vi "New Exchanges.vi"(8 "error in (no error)":errorcluster caption="entrée d'erreur (pas d'erreur)", 10 "initial dictionary (empty)":cluster{"key":variant, "value":variant}[](array[cluster]), 11 "Exchanges en entrée":refnum<class "Exchanges.lvclass"> caption="DNL_LabVIEW Object in") -> (0 "error out":errorcluster caption="sortie d'erreur", 3 "Exchanges en sortie":refnum<class "Exchanges.lvclass"> caption="DNL_LabVIEW Object out")   [LabVIEW 2012, in "Exchanges.lvclass"]
uses:
  Exchanges.lvclass
  Exchanges.lvclass/Exchanges.ctl
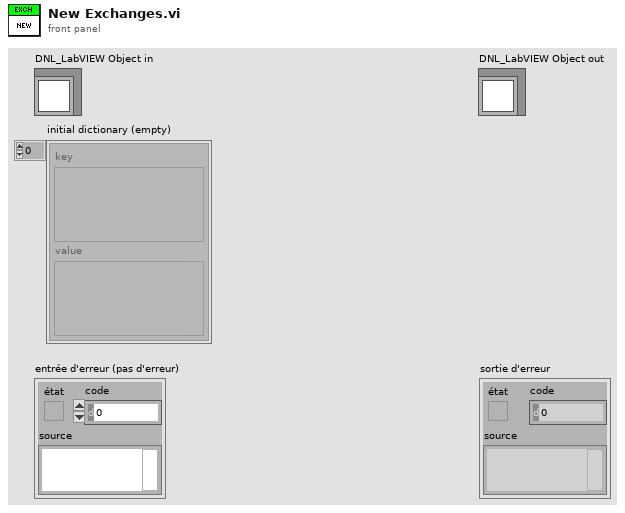
[diagram p1: front panel]
types:
  T1 = typedef "Dictionary Object RefNum__ogtk.ctl" = refnum<k1>
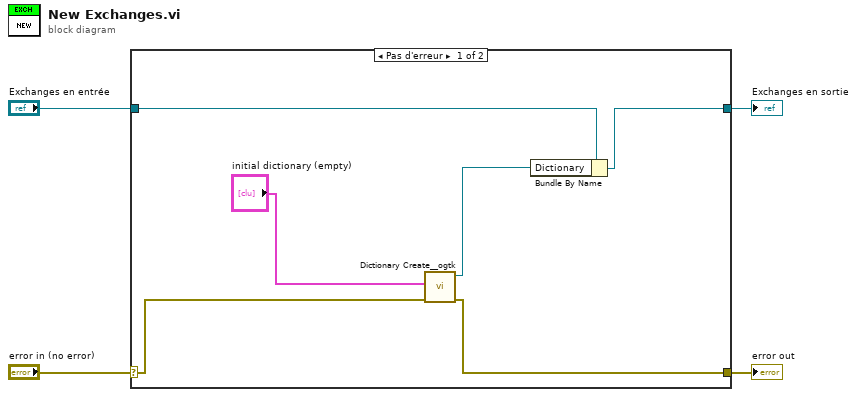
[diagram p0: block diagram]
diagram:
  n1 = case shown="Pas d'erreur" "error in (no error)" {
    selector: "error in (no error)" -> [w8 w12]
    tunnel: [w7 w12] -> w3
    tunnel: [w5 w11] -> w1
    tunnel: "Exchanges en entrée" -> [w6 w11]
    frame No Error {
      n2 = call <userlib>:"Dictionary Create__ogtk.vi"("error in (no error)"=w8, "initial dictionary (empty)"="initial dictionary (empty)") -> ("error out"=w7:errorcluster, "dictionary out"=w10:T1)  [unwired: 8 in]
      n3 = Bundle By Name(cluster=w6, "Dictionary"=w10) -> (w5:refnum<class "Exchanges.lvclass">)
    }
    frame Error {
    }
  }
  "error out" <- w3
  "Exchanges en sortie" <- w1
